vi "saveDataNodeBegin.vi"(8 "error in (no error)":errorcluster, 9 "indent":i32, 10 "XML Refnum in":refnum<file>, 11 "Categories in":refnum<class "Categories.lvclass">) -> (0 "error out":errorcluster, 2 "XML Refnum out":refnum<file>, 3 "Categories out":refnum<class "Categories.lvclass">)   [LabVIEW 2013, in "Categories.lvclass"]
doc: "Begins the process of saving a xceData Node to an XML formatted file."
uses:
  Categories.lvclass
  xCE/xceNode/xceNode.lvclass
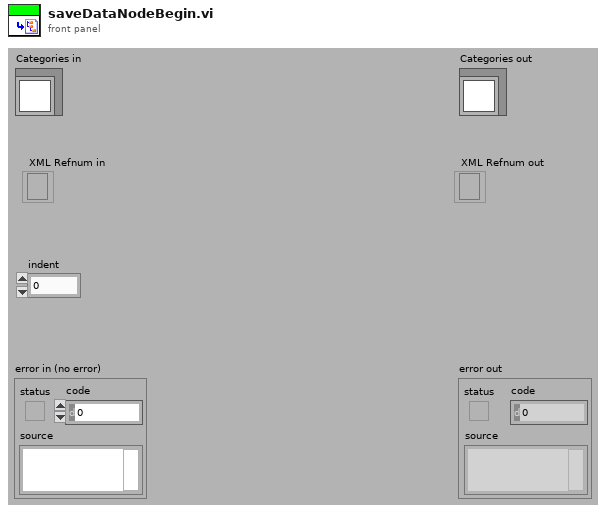
[diagram p1: front panel]
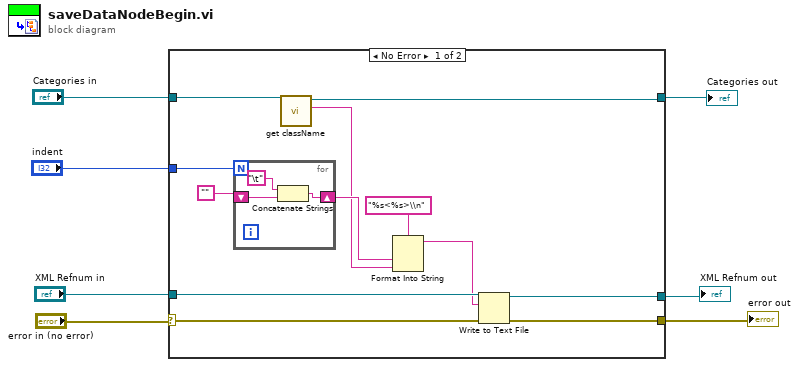
[diagram p0: block diagram]
diagram:
  n1 = case shown="No Error" "error in (no error)" {
    selector: "error in (no error)" -> [w12 w24]
    tunnel: "Categories in" -> [w15 w25]
    tunnel: "indent" -> [w18 _]
    tunnel: [w13 w25] -> w4
    tunnel: "XML Refnum in" -> [w11 w23]
    tunnel: [w10 w23] -> w2
    tunnel: [w9 w24] -> w1
    frame No Error {
      n2 = for {
        N: w18 -> [_]
        shift-right: [w22] -> w17
        shift-left: "" -> [w21]
        n3 = Concatenate Strings("\t", w21) -> (w22:string)
      }
      n4 = call "get className.vi"("xceNode in"=w15) -> ("Class name"=w14:string, "xceNode out"=w13:refnum<class "Categories.lvclass">)  [unwired: 8 in, 1 out]
      n5 = Format Into String(format string="%s<%s>\\n", w17, w14) -> (resulting string=w8:string)  [unwired: 2 in, 1 out]
      n6 = Write to Text File(file (use dialog)=w11, text=w8, error in=w12) -> (refnum out=w10:refnum<file>, error out=w9:errorcluster)  [unwired: 1 in, 1 out]
    }
    frame Error {
    }
  }
  "error out" <- w1
  "Categories out" <- w4
  "XML Refnum out" <- w2
